vi "ReadLimit.vi"(5 "Teleop Local Data In":T1 {"Vision"."Theta_Y" format="%.1f"; "Vision"."Theta_X" format="%.1f"; "Potentio" format="%.1f"; "Drive_Enc_R" format="%.1f"; "Drive_Enc_L" format="%.1f"; "Gyro_Angle" format="%.1f"; "Encoder_Lift" format="%.1f"; "Motor_Lift" format="%.3f"; "Motor_Intake" format="%.3f"; "Drive_Twist" format="%.3f"; "Drive_Forward" format="%.3f"}, 9 "error in":errorcluster) -> (6 "Teleop Local Data Out":T1 {"Vision"."Theta_Y" format="%.1f"; "Vision"."Theta_X" format="%.1f"; "Potentio" format="%.1f"; "Drive_Enc_R" format="%.1f"; "Drive_Enc_L" format="%.1f"; "Gyro_Angle" format="%.1f"; "Encoder_Lift" format="%.1f"; "Motor_Lift" format="%.3f"; "Motor_Intake" format="%.3f"; "Drive_Twist" format="%.3f"; "Drive_Forward" format="%.3f"}, 10 "error out":errorcluster)   [LabVIEW 2018]
uses:
  Typedefs/typedef_cluster_TeleOp_Local_Data.ctl
  Typedefs/typedef_cluster_Joystick.ctl
  Typedefs/typedef_cluster_Vision.ctl
  Typedefs/typedef_enum_refnums.ctl
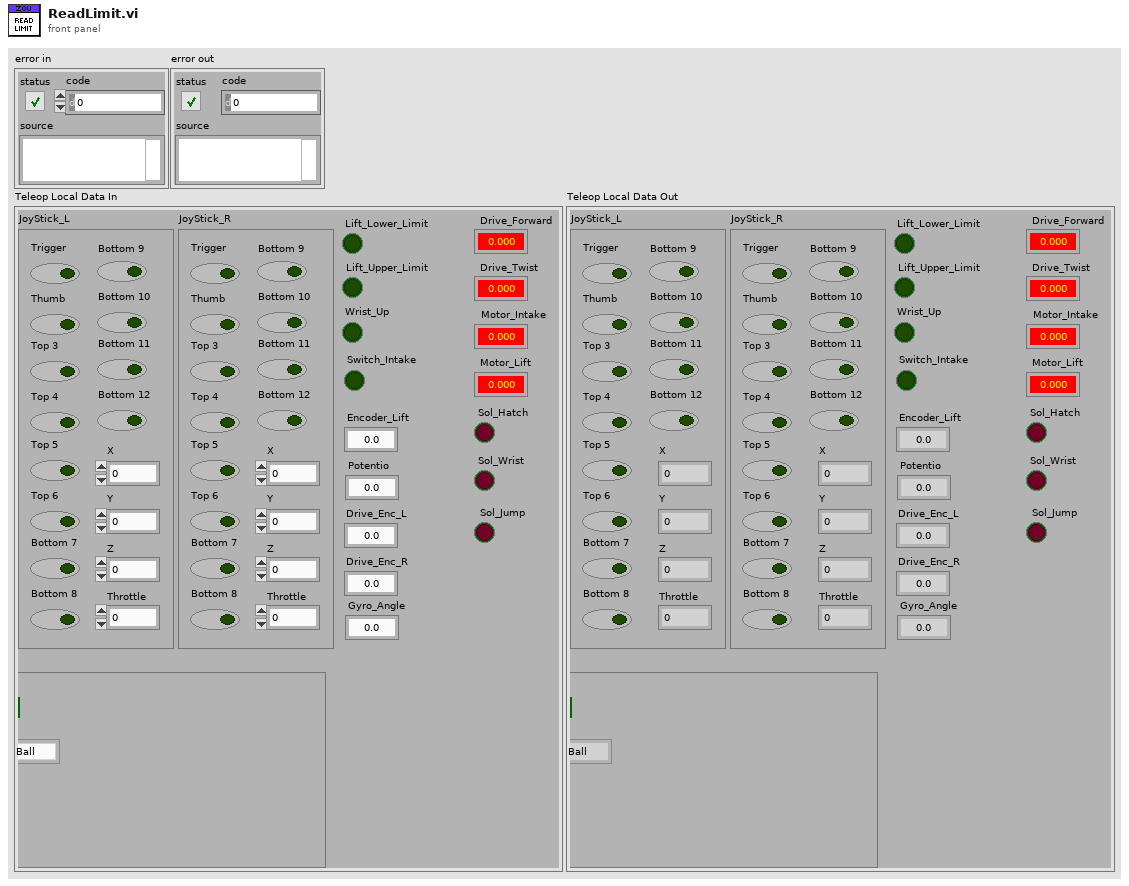
[diagram p1: front panel]
types:
  T1 = typedef "typedef_cluster_TeleOp_Local_Data.ctl" = cluster{"Lift_Lower_Limit":bool, "Wrist_Up":bool, "Switch_Intake":bool, "Encoder_Lift":dbl, "Sol_Wrist":bool, "Motor_Intake":dbl, "Motor_Lift":dbl, "Drive_Forward":dbl, "Drive_Twist":dbl, "Sol_Hatch":bool, "Gyro_Angle":dbl, "Drive_Enc_L":dbl, "Drive_Enc_R":dbl, "JoyStick_L":T2, "JoyStick_R":T2, "Potentio":dbl, "Vision":T3, "Lift_Upper_Limit":bool, "Sol_Jump":bool}
  T2 = typedef "typedef_cluster_Joystick.ctl" = cluster{"X":dbl, "Y":dbl, "Z":dbl, "Throttle":dbl, "Trigger":bool, "Thumb":bool, "Top 3":bool, "Top 4":bool, "Top 5":bool, "Top 6":bool, "Bottom 7":bool, "Bottom 8":bool, "Bottom 9":bool, "Bottom 10":bool, "Bottom 11":bool, "Bottom 12":bool}
  T3 = typedef "typedef_cluster_Vision.ctl" = cluster{"Theta_X":dbl, "Theta_Y":dbl, "Has_Target":bool, "Seek_Ball":bool, "Pipeline":enum16{"Ball", "Dual_Target", "Single_Target"}}
  T4 = typedef "typedef_enum_refnums.ctl" = enum16{"Joy_L", "Joy_R", "Drive_Motors", "Intake_Motor", "Wrist_Solenoid", "Hatch_Solenoid", "Compressor", "Lift_Motor", "Lift_Motor_2", "Gyro", "Drive_Enc_L", "Drive_Enc_R", "Lift_Lower_Limit", "Lift_Upper_Limit", "Ball_Switch", "Jump_Solenoid"}
  T5 = typedef "WPI_SwitchDevRef.ctl" = cluster{"DevStatus":errorcluster, "DIO Channel":T6, "CntIndex":T7, "Normally Closed":bool}
  T6 = typedef "FPGA_DIOChannel.ctl" = enum8{"DIO 0", "DIO 1", "DIO 2", "DIO 3", "DIO 4", "DIO 5", "DIO 6", "DIO 7", "DIO 8", "DIO 9", "DIO MXP 0", "DIO MXP 1", "DIO MXP 2", "DIO MXP 3", "DIO MXP 4", "DIO MXP 5", "DIO MXP 6", "DIO MXP 7", "DIO MXP 8", "DIO MXP 9", "DIO MXP 10", "DIO MXP 11", "DIO MXP 12", "DIO MXP 13", "DIO MXP 14", "DIO MXP 15", "SPI Port CS1", "SPI Port CS2", "SPI Port CS3", "SPI Port MISO", "SPI Port MOSI", "Invalid"}
  T7 = typedef "FPGA_CounterCtrSystemIndex.ctl" = enum8{"Ctr 0", "Ctr 1", "Ctr 2", "Ctr 3", "Ctr 4", "Ctr 5", "Ctr 6", "Ctr 7", "Invalid"}
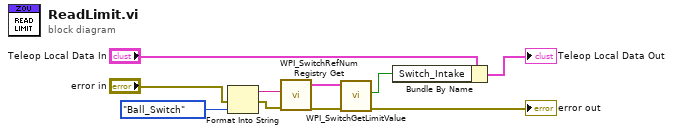
[diagram p0: block diagram]
diagram:
  n1 = Format Into String(error in="error in", typedef_enum_refnums."Ball_Switch" ("Enum")) -> (resulting string=w7:string, error out=w4:errorcluster)  [unwired: 2 in]
  n2 = call <vilib>:"WPI_SwitchRefNum Registry Get.vi"("error in (no error)"=w4, "refnum name"=w7) -> ("error out"=w9:errorcluster, "SwitchDevRef"=w10:T5)  [unwired: 8 in]
  n3 = call <vilib>:"WPI_SwitchGetLimitValue.vi"("error in (no error)"=w9, "SwitchDevRef"=w10) -> ("error out"=→"error out":errorcluster, "Switch Pressed"=w8:bool)  [unwired: 7 in, 1 out]
  n4 = Bundle By Name(cluster="Teleop Local Data In", "Switch_Intake"=w8) -> (→"Teleop Local Data Out":T1)
